vi "Score Particles.vi"(7 "Image Size":cluster{i32, i32}, 8 "Area Size Limit":i32=444, 9 "Particle Count Limit":i32=10, 10 "Image Dst":T2, 11 "Image Refnum in":T2) -> (2 "Targets":T1(array[cluster]), 3 "Image Refnum out":T2)   [LabVIEW 2011]
doc: "Score the largest particles in the image to determine how well they match the target attributes. Specifically, calculate how rectangular a particle is, inspect its aspect ratio, and determine if it is hollow (having pixels on around the edges, but off in the large center)."
uses:
  <vilib>/vision/Image Controls.llb/IMAQ Image.ctl
  <vilib>/vision/NI_Vision_Development_Module.lvlib
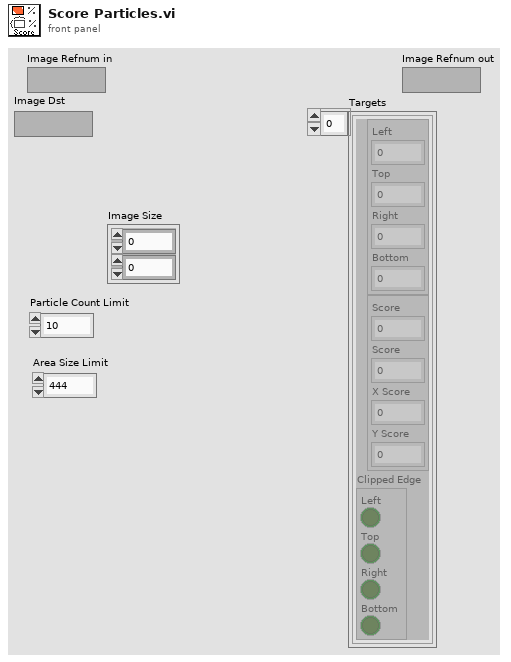
[diagram p1: front panel]
types:
  T1 = cluster{cluster{"Left":dbl, "Top":dbl, "Right":dbl, "Bottom":dbl}, cluster{"Score":dbl, "Score":dbl, "X Score":dbl, "Y Score":dbl}, "Clipped Edge":cluster{"Left":bool, "Top":bool, "Right":bool, "Bottom":bool}}[]
  T2 = typedef "IMAQ Image.ctl" = refnum<image>
  T3 = typedef "Particle Parameters" = i32
  T4 = typedef "Image Type" = u32
  T5 = cluster{"Left":dbl, "Top":dbl, "Right":dbl, "Bottom":dbl}
  T6 = cluster{"Left":bool, "Top":bool, "Right":bool, "Bottom":bool}
  T7 = cluster{"Score":dbl, "Score":dbl, "X Score":dbl, "Y Score":dbl}
  T8 = cluster{cluster{"Left":dbl, "Top":dbl, "Right":dbl, "Bottom":dbl}, cluster{"Score":dbl, "Score":dbl, "X Score":dbl, "Y Score":dbl}, "Clipped Edge":cluster{"Left":bool, "Top":bool, "Right":bool, "Bottom":bool}}
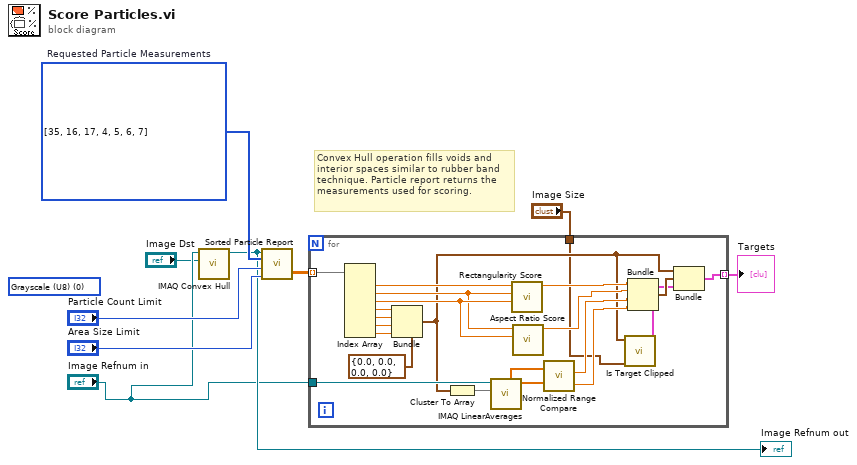
[diagram p0: block diagram]
diagram:
  w6 = T3[] [35, 16, 17, 4, 5, 6, 7] items=["Center of Mass X", "Center of Mass Y", "First Pixel X", "First Pixel Y", "Bounding Rect Left", "Bounding Rect Top", "Bounding Rect Right", "Bounding Rect Bottom", "Max Feret Diameter Start X", "Max Feret Diameter Start Y", "Max Feret Diameter End X", "Max Feret Diameter End Y", "Max Horiz. Segment Length Left", "Max Horiz. Segment Length Right", "Max Horiz. Segment Length Row", "-", "Bounding Rect Width", "Bounding Rect Height", "Bounding Rect Diagonal", "Perimeter", "Convex Hull Perimeter", "Holes' Perimeter", "Max Feret Diameter", "Equivalent Ellipse Major Axis", "Equivalent Ellipse Minor Axis", "Equivalent Ellipse Minor Axis (Feret)", "Equivalent Rect Long Side", "Equivalent Rect Short Side", "Equivalent Rect Diagonal", "Equivalent Rect Short Side (Feret)", "Average Horiz. Segment Length", "Average Vert. Segment Length", "Hydraulic Radius", "Waddel Disk Diameter", "-", "Area", "Holes' Area", "Particle & Holes' Area", "Convex Hull Area", "Image Area", "-", "Number of Holes", "Number of Horiz. Segments", "Number of Vert. Segments", "-", "Orientation", "Max Feret Diameter Orientation", "-", "% Area/Image Area", "% Area/(Particle & Holes' Area)", "Ratio of Equivalent Ellipse Axes", "Ratio of Equivalent Rect Sides", "-", "Elongation Factor", "Compactness Factor", "Heywood Circularity Factor", "Type Factor", "-", "Sum X", "Sum Y", "Sum XX", "Sum XY", "Sum YY", "Sum XXX", "Sum XXY", "Sum XYY", "Sum YYY", "-", "Moment of Inertia XX", "Moment of Inertia XY", "Moment of Inertia YY", "Moment of Inertia XXX", "Moment of Inertia XXY", "Moment of Inertia XYY", "Moment of Inertia YYY", "Norm. Moment of Inertia XX", "Norm. Moment of Inertia XY", "Norm. Moment of Inertia YY", "Norm. Moment of Inertia XXX", "Norm. Moment of Inertia XXY", "Norm. Moment of Inertia XYY", "Norm. Moment of Inertia YYY", "Hu Moment 1", "Hu Moment 2", "Hu Moment 3", "Hu Moment 4", "Hu Moment 5", "Hu Moment 6", "Hu Moment 7"]  # Requested Particle Measurements
  (unwired) T4 0 items=["Grayscale (U8)", "Grayscale (I16)", "Grayscale (SGL)", "Complex (CSG)", "RGB (U32)", "HSL (U32)", "RGB (U64)", "Grayscale (U16)"] ("Image Type")
  # "Convex Hull operation fills voids and\ninterior spaces similar to rubber band\ntechnique. Particle report returns the\nmeasurements used for scoring."
  n1 = call "IMAQ Convex Hull"("Image Dst"="Image Dst", "Image Src"="Image Refnum in") -> ("Image Dst Out"=w5:T2)  [unwired: 2 in, 7 out]
  "Image Refnum out" <- w5
  n2 = call "Sorted Particle Report.vi"("Area Size Limit"="Area Size Limit", "Particle Count Limit"="Particle Count Limit", "Pixel Measurements"=w6, "Image in"=w5) -> ("Sorted Data"=w9:dbl[][])  [unwired: 1 out]
  n3 = for {
    tunnel: [w29] -> w2 mode=indexing
    tunnel: "Image Refnum in" -> [w25]
    tunnel: w9 -> [w24] mode=indexing
    tunnel: "Image Size" -> [w10]
    n4 = Index Array(array=w24) -> (element #1=w30:dbl, element #2=w18:dbl, element #3=w19:dbl, element #4=w20:dbl, element #5=w21:dbl, element #6=w22:dbl, element #7=w23:dbl)  [unwired: 7 in]
    n5 = Bundle(cluster=T5 {"Left"=0.0, "Top"=0.0, "Right"=0.0, "Bottom"=0.0}, "Left"=w20, "Top"=w21, "Right"=w22, "Bottom"=w23) -> (w11:T5)
    n6 = Cluster To Array(cluster=w11) -> (array=w26:dbl[])
    n7 = call "IMAQ LinearAverages"("Optional Rectangle"=w26, "Image Src"=w25) -> ("Y Axis Averages"=w28:sgl[], "X Axis Averages"=w27:sgl[])  [unwired: 2 in, 6 out]
    n8 = call "Rectangularity Score.vi"("Height"=w19, "Width"=w18, "Area"=w30) -> ("Score"=w16:dbl)  [unwired: 8 in]
    n9 = call "Aspect Ratio Score.vi"("Height"=w19, "Width"=w18) -> ("Score"=w15:dbl)  [unwired: 9 in]
    n10 = call "Normalized Range Compare.vi"("Y Averages"=w28, "X Averages"=w27) -> ("Y Score"=w13:dbl, "X Score"=w14:dbl)
    n11 = call "Is Target Clipped.vi"("Image Size"=w10, "Bounding Box"=w11) -> ("Clipped Edge"=w12:T6)  [unwired: 9 in]
    n12 = Bundle("Score"=w16, "Score"=w15, "X Score"=w14, "Y Score"=w13) -> (w17:T7)  [unwired: 1 in]
    n13 = Bundle(w11, w17, "Clipped Edge"=w12) -> (w29:T8)  [unwired: 1 in]
  }
  "Targets" <- w2
